vi "Z6_Beamline_Chief.set i Attr and create DIM Services.vi"(0 "Refnum in":refnum<vi>, 5 "error in":errorcluster) -> (14 "i ref out":refnum<vi>, 17 "i Attr":T1={"R2S Service ID"=-1}, 19 "error out":errorcluster)   [LabVIEW 2014, in "Z6_Beamline_Chief.lvlib"]
doc: "This VI creates DIM services."
uses:
  Z6_Beamline_Chief.lvlib
  Z6_Beamline_Chief.i attribute.ctl
  PH_Common/PH_Common.lvlib
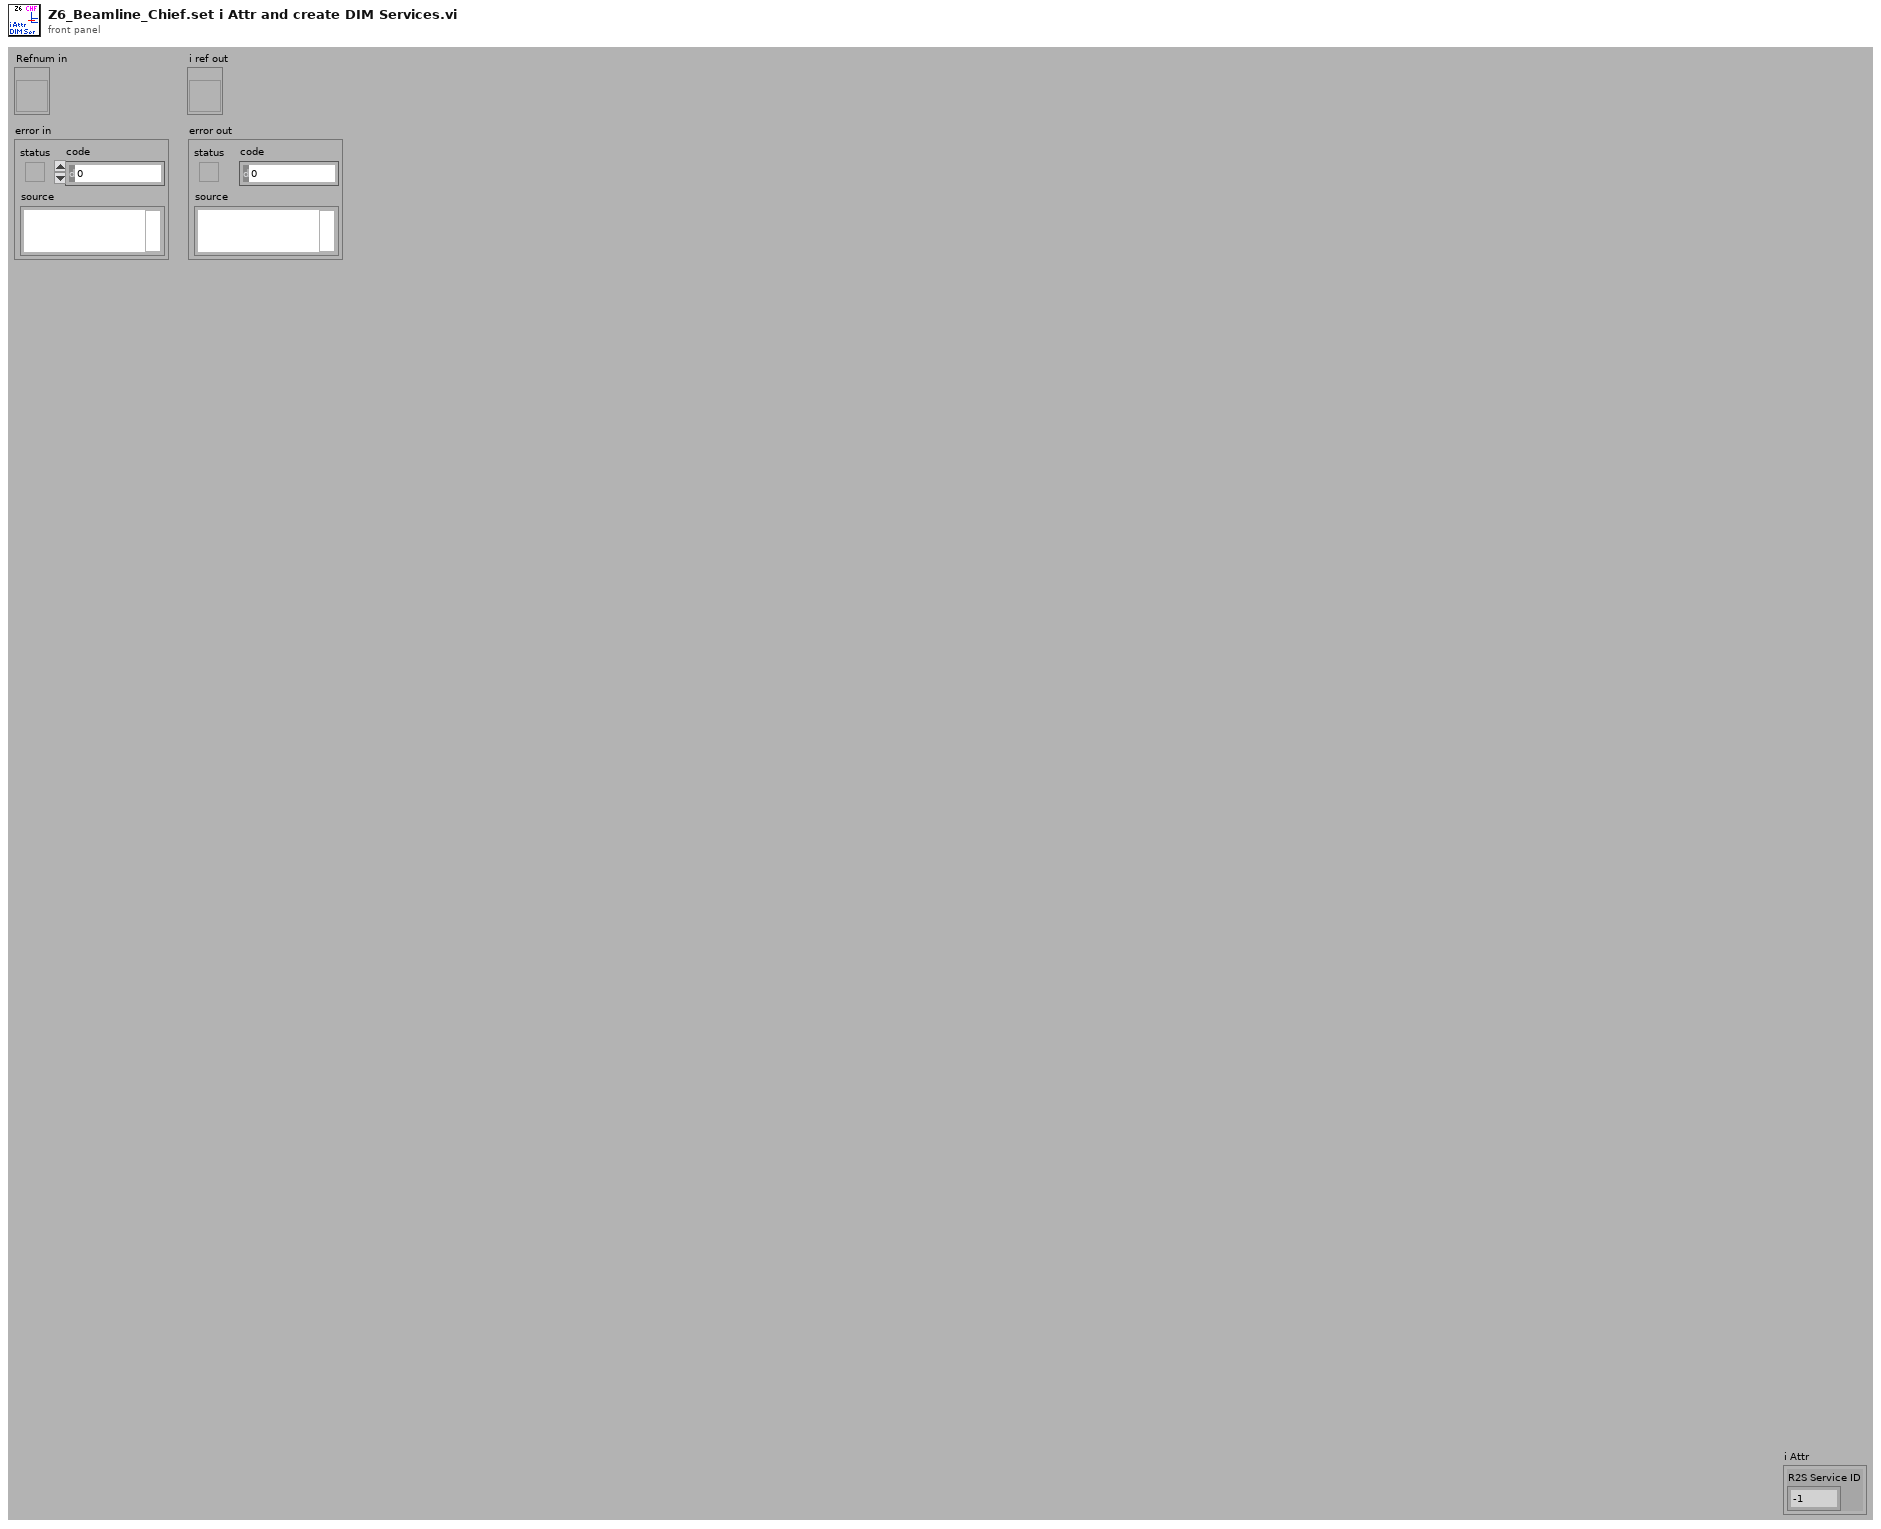
[diagram p1: front panel]
types:
  T1 = typedef "Z6_Beamline_Chief.lvlib/Z6_Beamline_Chief.i attribute.ctl" = cluster{"R2S Service ID":i32}
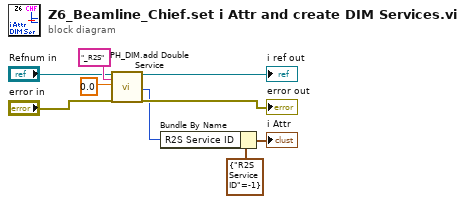
[diagram p0: block diagram]
diagram:
  n1 = call "PH_DIM.add Double Service.vi"("i ref in"="Refnum in", "Service Name"="_R2S" ("string"), "Double Value"=0.0 ("x"), "error in (no error)"="error in") -> ("i ref out"=→"i ref out":refnum<vi>, "Service ID"=w3:i32, "error out"=→"error out":errorcluster)  [unwired: 13 in]
  n2 = Bundle By Name(cluster=T1 {"R2S Service ID"=-1} ("i attribute"), "R2S Service ID"=w3) -> (→"i Attr":T1)
